vi "Spreadsheet Storage.vi"() -> ()   [LabVIEW 2015]
uses:
  <vilib>/Utility/file.llb/Write Delimited Spreadsheet (DBL).vi
panel:
  in  "Waveform Parameters":T1
  in  "Digitizing Parameters":T2
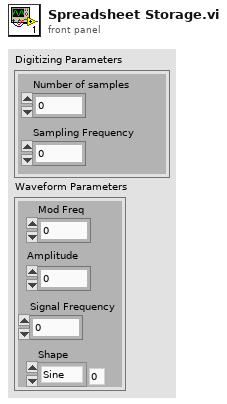
[diagram p1: front panel]
types:
  T1 = cluster{"Mod Freq":dbl, "Amplitude":dbl, "Shape":enum16{"Sine", "Cosine", "DC Level", "Square", "User Defined"}, "Signal Frequency":dbl}
  T2 = cluster{"Number of samples":dbl, "Sampling Frequency":dbl}
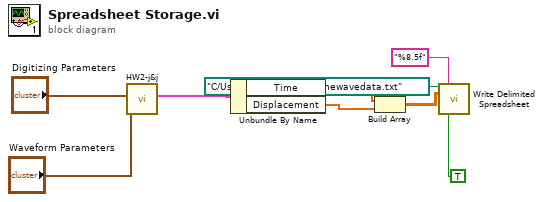
[diagram p0: block diagram]
diagram:
  n1 = call "HW2-j&j.vi"("AM Wave Parameters"="Waveform Parameters", "Digitizing Parameters"="Digitizing Parameters") -> ("AM Wave"=w9:cluster{"Time":dbl[], "Displacement":dbl[]})  [unwired: 9 in]
  n2 = Unbundle By Name(w9) -> ("Time"=w5:dbl[], "Displacement"=w4:dbl[])
  n3 = Build Array(w5, w4) -> (w3:dbl[][])
  n4 = call-poly <vilib>:"Write Delimited Spreadsheet.vi"("file path (dialog if empty)"=path "C:/Users/atchaj/week4/sinewavedata.txt", "format (%.3f)"="%8.5f", "2D data"=w3, "transpose? (F)"=TRUE) -> ()  [unwired: 10 in, 2 out]
